vi "AudioStreamer.Get Config.vi"() -> (0 "config":T1)   [LabVIEW 2020]
uses:
  Typedefs/AudioStreamer.Config Return Data.ctl
  Typedefs/AudioStreamer.Globals.vi
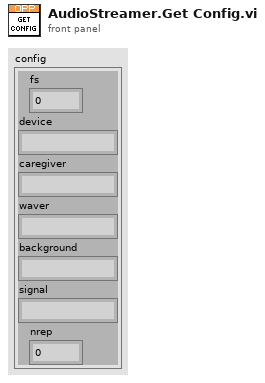
[diagram p1: front panel]
types:
  T1 = typedef "AudioStreamer.Config Return Data.ctl" = cluster{"fs":dbl, "device":string, "caregiver":string, "waver":string, "background":string, "signal":string, "nrep":i32}
  T2 = typedef "AudioStreamer.Config.ctl" = cluster{"Fs (Hz)":dbl, "output":string, "mic":string, "nrep":i32, "caregiver":cluster{"name":string, "data":sgl[]}, "waver":cluster{"name":string, "data":sgl[]}, "background":cluster{"name":string, "data":sgl[]}, "signal":cluster{"name":string, "data":sgl[]}}
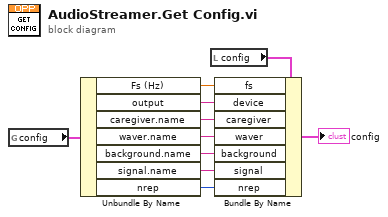
[diagram p0: block diagram]
diagram:
  n1 = global read "AudioStreamer.Globals.vi" "config"() -> (w10:T2)
  n2 = Unbundle By Name(w10) -> ("Fs (Hz)"=w7:dbl, "output"=w6:string, "caregiver.name"=w5:string, "waver.name"=w4:string, "background.name"=w3:string, "signal.name"=w2:string, "nrep"=w1:i32)
  n3 = local read "config"() -> (w8:T1)
  n4 = Bundle By Name(cluster=w8, "fs"=w7, "device"=w6, "caregiver"=w5, "waver"=w4, "background"=w3, "signal"=w2, "nrep"=w1) -> (→"config":T1)
